vi "Update Label.vi"(8 "error in (no error)":errorcluster, 9 "Actor's Label":string, 10 "Actor's Self Q":refnum<class "Message Enqueuer.lvclass">, 11 "Actor Monitor New in":refnum<class "Actor Monitor.lvclass">) -> (0 "error out":errorcluster, 3 "Actor Monitor New out":refnum<class "Actor Monitor.lvclass">)   [LabVIEW 2020, in "Monitored Actor.lvlib" / "Actor Monitor.lvclass"]
doc: "Updates the actor's label\n\nCopyright: MGI 2016\nAuthor: Derek Trepanier"
uses:
  <vilib>/MGI/Monitored Actor/Actor Monitor/Actor Monitor/Actor Monitor.lvclass
  <vilib>/ActorFramework/Message Enqueuer/Message Enqueuer.lvclass
  <vilib>/MGI/Monitored Actor/Actor Monitor/Actor Monitor/Actor Monitor.lvclass/Actor Monitor.ctl
  <vilib>/MGI/Monitored Actor/Monitor Data/Monitor Data.lvclass
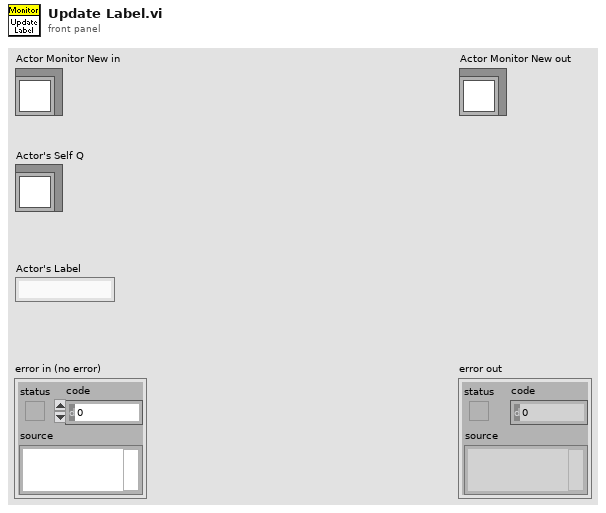
[diagram p1: front panel]
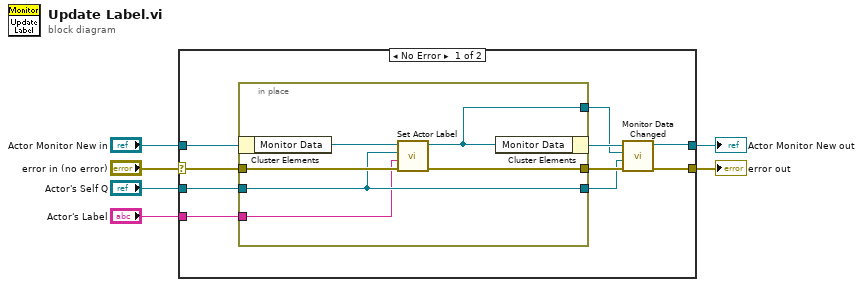
[diagram p0: block diagram]
diagram:
  n1 = case shown="No Error" "error in (no error)" {
    selector: "error in (no error)" -> [w14 w24]
    tunnel: [w11 w24] -> w5
    tunnel: [w9 w23] -> w3
    tunnel: "Actor Monitor New in" -> [w16 w23]
    tunnel: "Actor's Self Q" -> [w13 _]
    tunnel: "Actor's Label" -> [w12 _]
    frame No Error {
      n2 = in-place {
        in-place-border: [w21] -> w15
        in-place-border: w14 -> [w20]
        in-place-border: w13 -> [w18]
        in-place-border: w12 -> [w17]
        in-place-border: [w19] -> w8
        in-place-border: [w18] -> w7
        n3 = in-place-cluster #1(w16) -> ("Monitor Data"=w22:refnum<class "Monitor Data.lvclass">)
        n4 = call <vilib>:"Set Actor Label.vi"("error in (no error)"=w20, "Actor Label"=w17, "Actor's Self Q"=w18, "Monitor Data in"=w22) -> ("error out"=w21:errorcluster, "Monitor Data out"=w19:refnum<class "Monitor Data.lvclass">)  [unwired: 6 in]
        n5 = in-place-cluster #1("Monitor Data"=w19) -> (w10:refnum<class "Actor Monitor.lvclass">)
      }
      n6 = call-dynamic "Monitor Data Changed.vi"("error in (no error)"=w15, "Changed Actor's Q"=w7, "Monitor Data"=w8, "Actor Monitor New in"=w10) -> ("error out"=w11:errorcluster, "Actor Monitor New out"=w9:refnum<class "Actor Monitor.lvclass">)  [unwired: 6 in]
    }
    frame Error {
    }
  }
  "error out" <- w5
  "Actor Monitor New out" <- w3
